vi "CLEventPlayback.vi"() -> ()   [LabVIEW 2017]
uses:
  <vilib>/DAQmx/read.llb/DAQmx Read (Counter U32 1Chan 1Samp).vi
  <vilib>/DAQmx/write.llb/DAQmx Write (Analog Wfm 1Chan NSamp).vi
  <vilib>/DAQmx/miscellaneous.llb/DAQmx Fill In Error Info.vi
panel:
  in  "Sham stim AO channel":tag="pciDAQ/ao2"
  in  "Events file":path
  in  "OEP sample clock in":tag="/pciDAQ/PFI0"
  in  "Onboard counter":tag="pciDAQ/ctr0"
  in  "Real stim AO channel":tag="pciDAQ/ao0"
  in  "OEP stim/sham TTL chans":u16[](array[numeric])=[2, 3] caption="probe channel" min=1 max=8
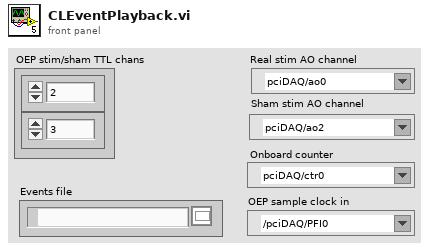
[diagram p1: front panel]
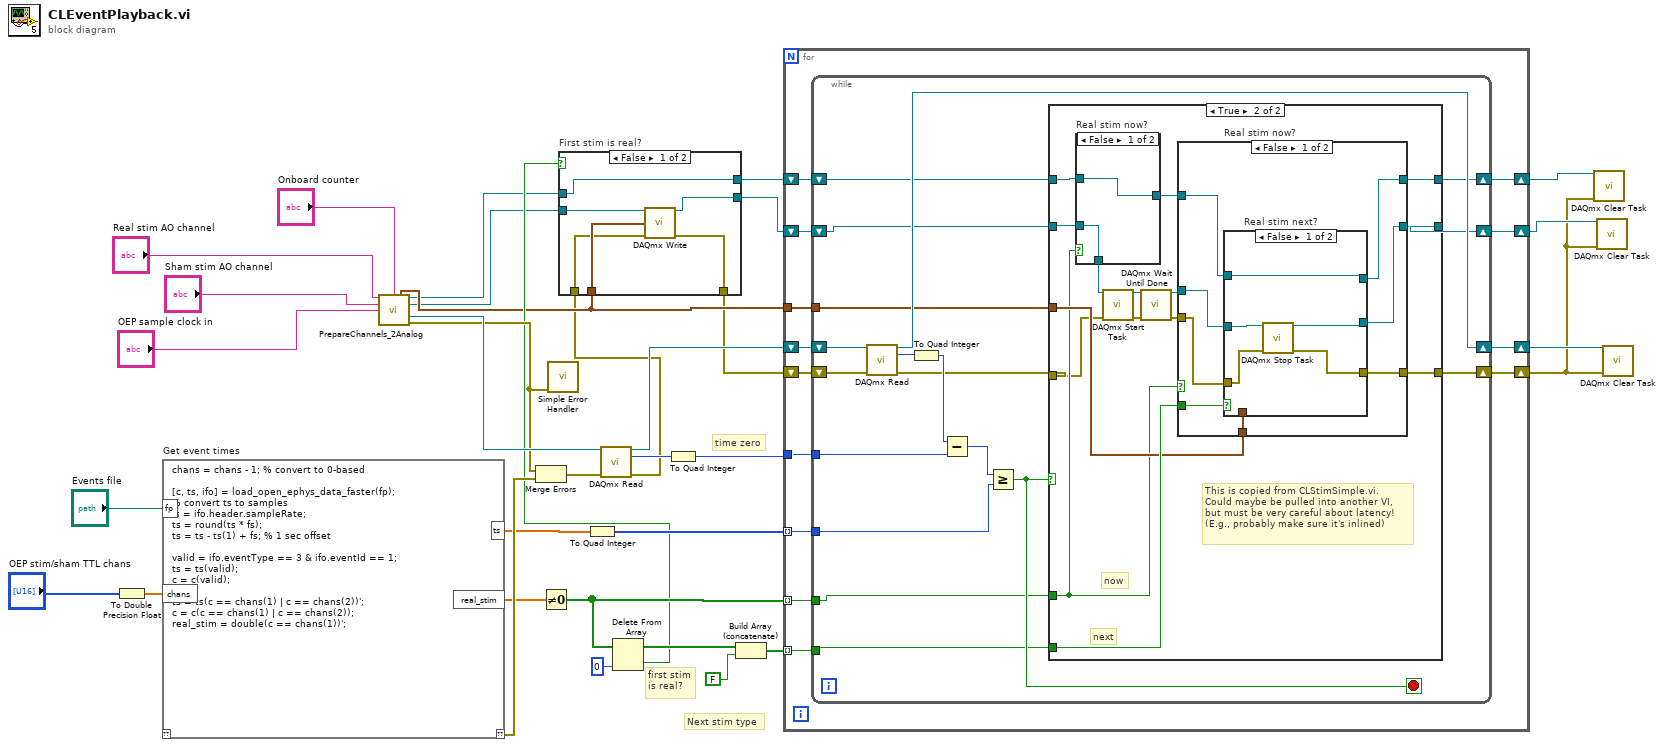
[diagram p0: block diagram]
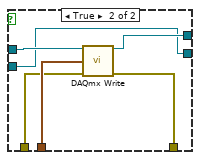
[diagram p2: hidden frame]
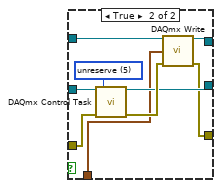
[diagram p5: hidden frame]
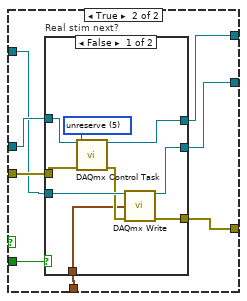
[diagram p6: hidden frame]
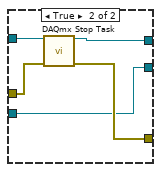
[diagram p7: hidden frame]
diagram:
  # "first stim\nis real?"
  # "Next stim type"
  # "time zero"
  n1 = To Double Precision Float(number="OEP stim/sham TTL chans") -> (double precision float=w32:dbl[])
  n2 = script code="chans = chans - 1; % convert to 0-based\n\n[c, ts, ifo] = load_open_ephys_data_faster(fp);\n% convert ts to samples\nfs = ifo.header.sampleRate;\nts = round(ts * fs);\nts = ts - ts(1) + fs; % 1 sec offset\n\nvalid = ifo.eventType == 3 & ifo.eventId == 1;\nts = ts(valid);\nc = c(valid);\n\nts = ts(c == chans(1) | c == chans(2))';\nc = c(c == chans(1) | c == chans(2));\nreal_stim = double(c == chans(1))';" "Get event times"("fp"="Events file", "chans"=w32) -> ("??"=w23:errorcluster, "ts"=w22:dbl[], "real_stim"=w12:dbl[])  [unwired: 1 in]
  n3 = call "PrepareChannels_2Analog.vi"("Real stim channel"="Real stim AO channel", "Onboard counter"="Onboard counter", "Sham stim channel"="Sham stim AO channel", "OEP sample clock in"="OEP sample clock in") -> ("Waveform Graph"=w7:waveform(dbl), "Real stim task"=w6:refnum<k21>, "Sham stim task"=w5:refnum<k21>, "ctr task out"=w14:refnum<k21>, "Error out"=w13:errorcluster)  [unwired: 7 in]
  n4 = Merge Errors(w13, w23) -> (w24:errorcluster)
  n5 = Not Equal To 0?(x=w12) -> (x != 0?=w10:bool[])
  n6 = call <vilib>:"Simple Error Handler.vi"("error in (no error)"=w13) -> ()  [unwired: 4 in, 5 out]
  n7 = To Quad Integer(1:w22) -> (0:w30:i64[])
  n8 = call-poly <vilib>:"DAQmx Read.vi"("task/channels in"=w14, "error in"=w24) -> ("task out"=w31:refnum<k21>, "data"=w29:u32, "error out"=w3:errorcluster)  [unwired: 11 in]
  n9 = Delete From Array(array=w10, index=0) -> (deleted portion=w8:bool, array with subset deleted=w9:bool[])  [unwired: 1 in]
  n10 = case "First stim is real?" shown="False" w8 {
    tunnel: w7 -> [w40 w46]
    tunnel: w6 -> [w37 w45]
    tunnel: w5 -> [w39 w41]
    tunnel: [w37 w44] -> w4
    tunnel: w3 -> [w36 w43]
    tunnel: [w35 w42] -> w2
    tunnel: [w38 w41] -> w1
    frame False {
      n11 = call-poly <vilib>:"DAQmx Write.vi"("task/channels in"=w39, "data"=w40, "error in"=w36) -> ("task out"=w38:refnum<k21>, "error out"=w35:errorcluster)  [unwired: 10 in, 1 out]
    }
    frame True {
      n12 = call-poly <vilib>:"DAQmx Write.vi"("task/channels in"=w45, "data"=w46, "error in"=w43) -> ("task out"=w44:refnum<k21>, "error out"=w42:errorcluster)  [unwired: 10 in, 1 out]
    }
  }
  n13 = To Quad Integer(1:w29) -> (0:w28:i64)
  n14 = Build Array (concatenate)(w9, FALSE) -> (w20:bool[])
  n15 = for {
    tunnel: w10 -> [w54] mode=indexing
    tunnel: w28 -> [w55]
    shift-right: [w57] -> w25
    shift-left: w31 -> [w59]
    shift-right: [w56] -> w19
    shift-left: w2 -> [w58]
    tunnel: w30 -> [w53] mode=indexing
    shift-right: [w50] -> w27
    shift-left: w4 -> [w52]
    shift-right: [w49] -> w26
    shift-left: w1 -> [w51]
    tunnel: w20 -> [w48] mode=indexing
    tunnel: w7 -> [w47]
    n16 = while {
      shift-right: [w75] -> w57
      shift-left: w59 -> [w77]
      shift-right: [w60] -> w56
      shift-left: w58 -> [w76]
      tunnel: w55 -> [w74]
      tunnel: w54 -> [w68]
      tunnel: w53 -> [w70]
      shift-right: [w65] -> w50
      shift-left: w52 -> [w67]
      shift-right: [w64] -> w49
      shift-left: w51 -> [w66]
      tunnel: w48 -> [w63]
      tunnel: w47 -> [w62]
      stop <- w69 stop-if-true
      n17 = call-poly <vilib>:"DAQmx Read.vi"("task/channels in"=w77, "error in"=w76) -> ("task out"=w75:refnum<k21>, "data"=w73:u32, "error out"=w61:errorcluster)  [unwired: 11 in]
      n18 = To Quad Integer(1:w73) -> (0:w72:i64)
      n19 = Subtract(x=w72, y=w74) -> (x-y=w71:i64)
      n20 = Greater Or Equal?(x=w71, y=w70) -> (x >= y?=w69:bool)
      n21 = case shown="True" w69 {
        tunnel: w68 -> [_ w90]
        tunnel: w67 -> [w80 w89]
        tunnel: w61 -> [w78 w87]
        tunnel: w66 -> [w79 w88]
        tunnel: [w80 w93] -> w65
        tunnel: [w79 w91] -> w64
        tunnel: w63 -> [_ w95]
        tunnel: w62 -> [_ w94]
        tunnel: [w78 w92] -> w60
        frame False {
        }
        frame True {
          # "next"
          # "now"
          # "This is copied from CLStimSimple.vi.\nCould maybe be pulled into another VI,\nbut must be very careful about latency!\n(E.g., probably make sure it's inlined)"
          n22 = case "Real stim now?" shown="False" w90 {
            tunnel: w89 -> [w96 w99]
            tunnel: w88 -> [w97 w98]
            tunnel: [w97 w99] -> w86
            tunnel: [w96 w98] -> w81
            frame False {
            }
            frame True {
            }
          }
          n23 = call <vilib>:"DAQmx Start Task.vi"("task/channels in"=w86, "error in"=w87) -> ("task out"=w85:refnum<k21>, "error out"=w84:errorcluster)  [unwired: 12 in]
          n24 = call <vilib>:"DAQmx Wait Until Done.vi"("task/channels in"=w85, "error in"=w84) -> ("task out"=w82:refnum<k21>, "error out"=w83:errorcluster)  [unwired: 12 in]
          n25 = case "Real stim now?" shown="False" w90 {
            tunnel: w94 -> [w106 w129]
            tunnel: w82 -> [w103 w123]
            tunnel: w81 -> [w104 w122]
            tunnel: [w101 w128] -> w93
            tunnel: [w107 w127] -> w92
            tunnel: [w100 w126] -> w91
            tunnel: w95 -> [w105 w125]
            tunnel: w83 -> [w102 w124]
            frame False {
              n26 = case "Real stim next?" shown="False" w105 {
                tunnel: w104 -> [w108 w116]
                tunnel: w103 -> [w112 w121]
                tunnel: w102 -> [w111 w120]
                tunnel: [w110 w115] -> w107
                tunnel: [w109 w117] -> w100
                tunnel: [w108 w114] -> w101
                tunnel: w106 -> [_ w113]
                frame False {
                  n27 = call <vilib>:"DAQmx Stop Task.vi"("task/channels in"=w112, "error in"=w111) -> ("task out"=w109:refnum<k21>, "error out"=w110:errorcluster)  [unwired: 12 in]
                }
                frame True {
                  w119 = 5 items=["verify"=2, "reserve"=4, "commit"=3, "unreserve"=5, "abort"=6] ("action")
                  n28 = call <vilib>:"DAQmx Control Task.vi"("task/channels in"=w121, "action"=w119, "error in"=w120) -> ("task out"=w117:refnum<k21>, "error out"=w118:errorcluster)  [unwired: 11 in]
                  n29 = call-poly <vilib>:"DAQmx Write.vi"("task/channels in"=w116, "data"=w113, "error in"=w118) -> ("task out"=w114:refnum<k21>, "error out"=w115:errorcluster)  [unwired: 10 in, 1 out]
                }
              }
            }
            frame True {
              n30 = case "Real stim next?" shown="False" w125 {
                tunnel: w129 -> [w133 _]
                tunnel: w122 -> [w135 w140]
                tunnel: w123 -> [w138 w143]
                tunnel: w124 -> [w136 w142]
                tunnel: [w132 w139] -> w128
                tunnel: [w131 w141] -> w127
                tunnel: [w130 w140] -> w126
                frame False {
                  w137 = 5 items=["verify"=2, "reserve"=4, "commit"=3, "unreserve"=5, "abort"=6] ("action")
                  n31 = call <vilib>:"DAQmx Control Task.vi"("task/channels in"=w138, "action"=w137, "error in"=w136) -> ("task out"=w132:refnum<k21>, "error out"=w134:errorcluster)  [unwired: 11 in]
                  n32 = call-poly <vilib>:"DAQmx Write.vi"("task/channels in"=w135, "data"=w133, "error in"=w134) -> ("task out"=w130:refnum<k21>, "error out"=w131:errorcluster)  [unwired: 10 in, 1 out]
                }
                frame True {
                  n33 = call <vilib>:"DAQmx Stop Task.vi"("task/channels in"=w143, "error in"=w142) -> ("task out"=w139:refnum<k21>, "error out"=w141:errorcluster)  [unwired: 12 in]
                }
              }
            }
          }
        }
      }
    }
  }
  n34 = call <vilib>:"DAQmx Clear Task.vi"("task in"=w27, "error in"=w19) -> ()  [unwired: 13 in, 1 out]
  n35 = call <vilib>:"DAQmx Clear Task.vi"("task in"=w26, "error in"=w19) -> ()  [unwired: 13 in, 1 out]
  n36 = call <vilib>:"DAQmx Clear Task.vi"("task in"=w25, "error in"=w19) -> ()  [unwired: 13 in, 1 out]
